vi "DSF.Engine.BuilderManager.Initialize Status Structures.vi"(8 "error in (no error)":errorcluster, 10 "number of builders":u64=1, 11 "Builder Manager in":refnum<class "DSF.Engine.BuilderManager.lvclass">) -> (0 "error out":errorcluster, 3 "Builder Manager out":refnum<class "DSF.Engine.BuilderManager.lvclass">)   [LabVIEW 2016, in "DSF.Engine.lvlib" / "DSF.Engine.BuilderManager.lvclass"]
uses:
  DSF.Engine.BuilderManager.lvclass
  Status/Status.Builder.State.lvclass
  C:/Git/Sourcetree/DSF/Source/Submodules/Memory/Source/Classes/Pointer/Memory.Pointer.lvclass
  DSF.Engine.BuilderManager.lvclass/DSF.Engine.BuilderManager.ctl
  Submodules/Memory/Source/Classes/Pointer/Memory.Pointer.New.1B.vi
  Submodules/Memory/Source/Classes/Pointer/Memory.Pointer.Allocate.vi
  Submodules/Memory/Source/Classes/Pointer/Memory.Pointer.lvclass
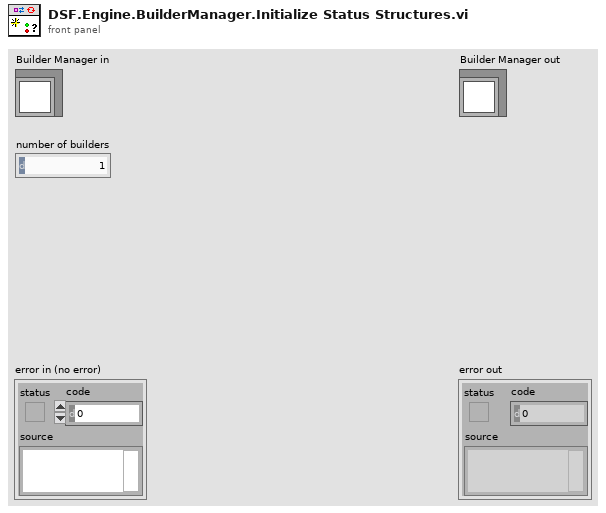
[diagram p1: front panel]
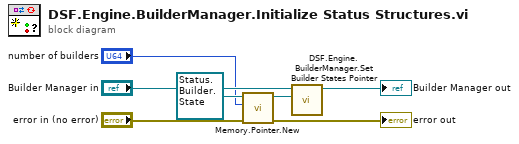
[diagram p0: block diagram]
diagram:
  n1 = call-poly "Memory.Pointer.New.vi"("error in (no error)"="error in (no error)", "count (1)"="number of builders", "pointer type"=refnum<class "Status.Builder.State.lvclass"> refnum ("Builder State in")) -> ("error out"=→"error out":errorcluster, "pointer out"=w3:refnum<class "Status.Builder.State.lvclass">)  [unwired: 7 in]
  n2 = call "DSF.Engine.BuilderManager.Set Builder States Pointer.vi"("Builder States"=w3, "Builder Manager in"="Builder Manager in") -> ("Builder Manager out"=→"Builder Manager out":refnum<class "DSF.Engine.BuilderManager.lvclass">)  [unwired: 9 in]
